vi "createConnection.vi"(8 "error in (no error)":errorcluster, 11 "OvenController in":refnum<class "OvenController.lvclass">) -> (0 "error out":errorcluster, 2 "IDeviceConnection":refnum<class "IDeviceConnection.lvclass">, 3 "OvenController out":refnum<class "OvenController.lvclass">)   [LabVIEW 2023, in "OvenController.lvclass"]
doc: "This is the Factory Method definition."
uses:
  OvenController.lvclass
  IDeviceConnection/IDeviceConnection.lvclass
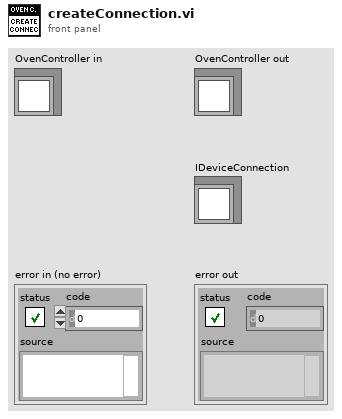
[diagram p1: front panel]
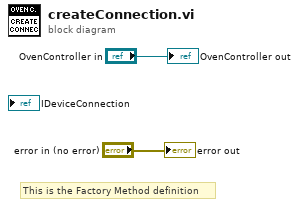
[diagram p0: block diagram]
diagram:
  # "This is the Factory Method definition"
  "error out" <- "error in (no error)"
  "OvenController out" <- "OvenController in"
